vi "QR Code_Import Image File.vi"(8 "error in":errorcluster, 9 "Load Color Palette? (F)":bool, 10 "File Path":path, 11 "Buffer Data In":T1) -> (0 "error out":errorcluster, 3 "Buffer Data Out":T1)   [LabVIEW 2016]
uses:
  Data Def/QR Code_Buffer Data.ctl
  <vilib>/vision/Image Controls.llb/IMAQ Image.ctl
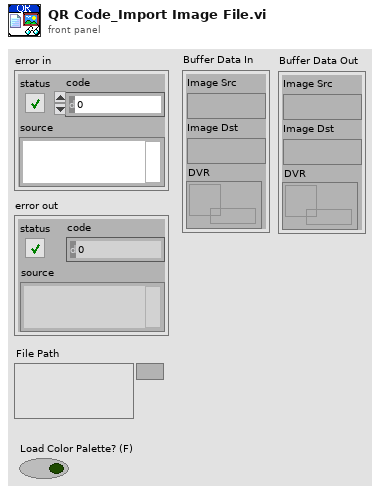
[diagram p1: front panel]
types:
  T1 = typedef "QR Code_Buffer Data.ctl" = cluster{"Image Src":T2, "Image Dst":T2, "DVR":refnum<data-value>}
  T2 = typedef "IMAQ Image.ctl" = refnum<image>
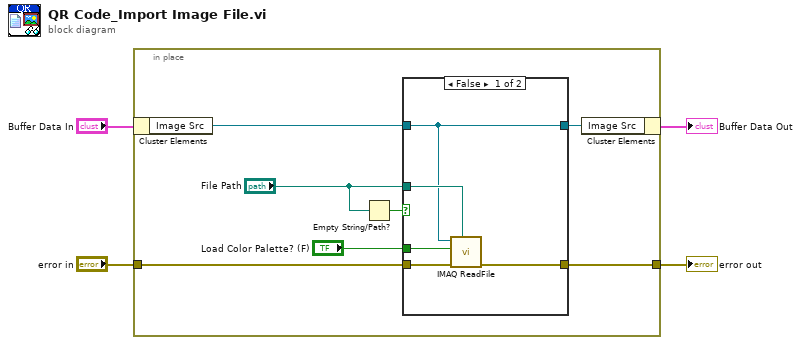
[diagram p0: block diagram]
diagram:
  n1 = in-place {
    in-place-border: "error in" -> [w11]
    in-place-border: [w8] -> w1
    n2 = in-place-cluster #1("Buffer Data In") -> ("Image Src"=w9:T2)
    n3 = Empty String/Path?(string/path="File Path") -> (empty?=w6:bool)
    n4 = case shown="False" w6 {
      tunnel: w11 -> [w16 w17]
      tunnel: "Load Color Palette? (F)" -> [w15 _]
      tunnel: w9 -> [w12 w18]
      tunnel: [w14 w17] -> w8
      tunnel: "File Path" -> [w13 _]
      tunnel: [w12 w18] -> w5
      frame False {
        n5 = call "IMAQ ReadFile"("File Path"=w13, "error in (no error)"=w16, "Load Color Palette? (No)"=w15, "Image"=w12) -> ("error out"=w14:errorcluster)  [unwired: 3 in, 4 out]
      }
      frame True {
      }
    }
    n6 = in-place-cluster #1("Image Src"=w5) -> (→"Buffer Data Out":T1)
  }
  "error out" <- w1
